vi "dll Main.vi"() -> ()   [LabVIEW 2018]
doc: "This template is for the Queued Message Handler design pattern.\n\nThe Event Handling Loop generates messages based on user interface actions.\n\nThe Message Handling Loop processes messages generated by the Event Handling Loop, or by other messages. The messages are string values, so new messages can be added easily to the Message Cases case structure in the Message Handling Loop. Each message cluster can also provide an optional value for Message Data, which is a variant that can be converted to whatever message-specific data is required."
uses:
  controls/dll UI Data.ctl
  support/Message Queue/dll Message Queue.lvlib
  <vilib>/Utility/error.llb/Error Cluster From Error Code.vi
  support/User Event - Stop/dll User Event - Stop.lvlib
  support/Message Queue/Enqueue Message (Single).vi
  <vilib>/ErrorRing/Error Ring.xnode
  C:/Users/booko/Desktop/ENABLE/UpDownCounter/bin/Debug/netstandard2.0/UpDownCounter.dll
  UpDownCounter/bin/Debug/netstandard2.0/UpDownCounter.dll
panel:
  out "Display <Replace Me>":string
  in  "Count Down":bool
  in  "Count Up":bool
  in  "Exit":bool
  # "These controls have associated \"Value Changed\" events configured in the Event Structure on the diagram.\n\nReplace them (and reconfigure the Event Structure) with the controls you need for your application."
  # "This template is for the Queued Message Handler design pattern.\n\nSee the block diagram for more information on how to use this template."
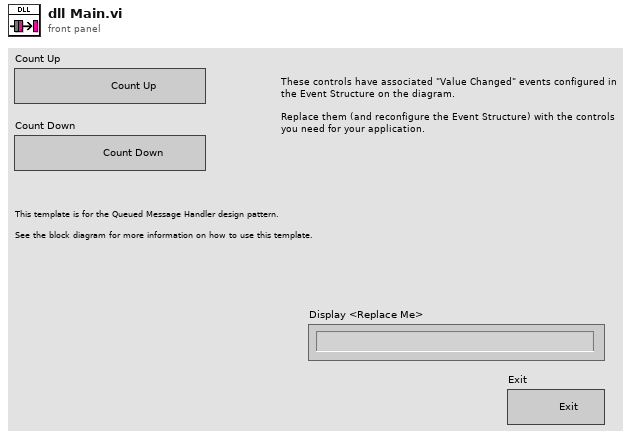
[diagram p1: front panel]
types:
  T1 = typedef "dll UI Data.ctl" = cluster{"Boolean <Replace Me>":bool, "String <Replace Me>":string, "Numeric <Replace Me>":dbl, "Do Something Ref":refnum<vi>, "Do Something Else Ref":refnum<vi>, "Data Display Ref":refnum<vi>, "Exit Button Ref":refnum<vi>, "UpDownCounterClass Reference":refnum<k24>}
  T2 = typedef "dll Message Queue.lvlib/All Message Queues.ctl" = cluster{"UI":refnum<queue>}
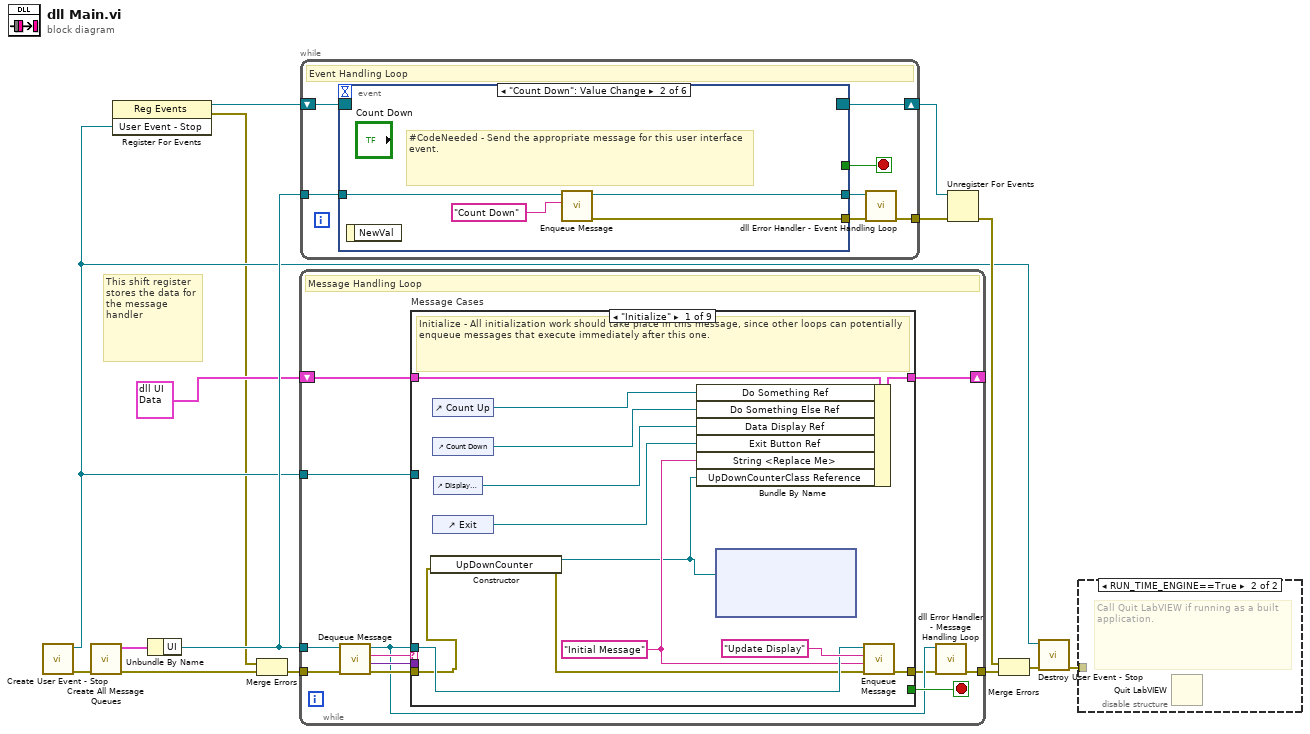
[diagram p0: block diagram]
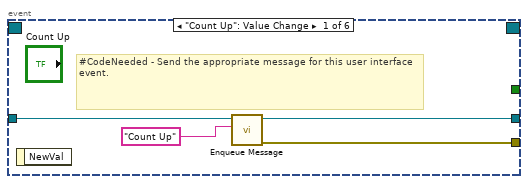
[diagram p3: hidden frame]
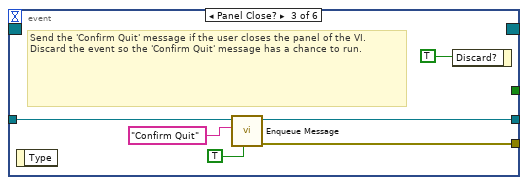
[diagram p4: hidden frame]
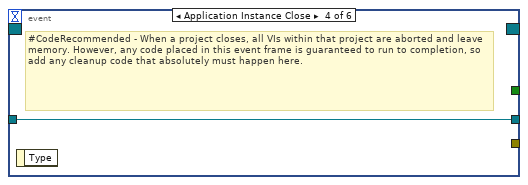
[diagram p5: hidden frame]
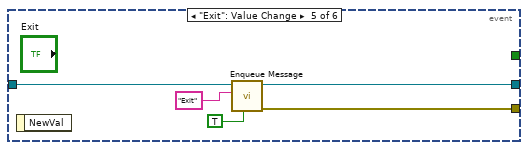
[diagram p6: hidden frame]
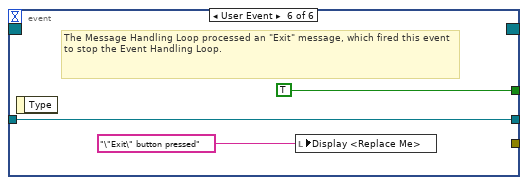
[diagram p7: hidden frame]
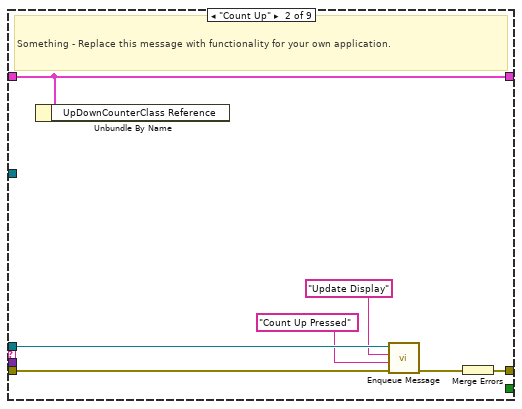
[diagram p8: hidden frame]
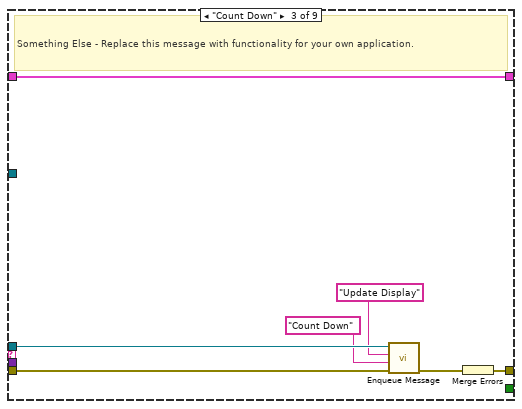
[diagram p9: hidden frame]
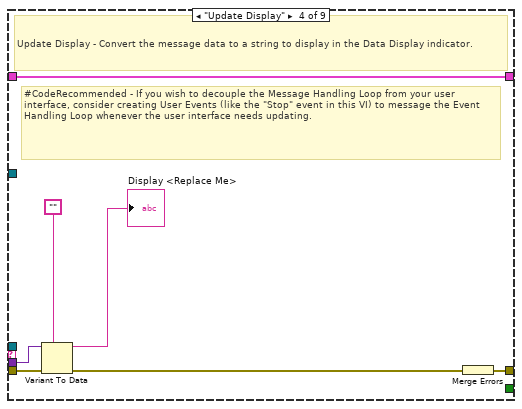
[diagram p10: hidden frame]
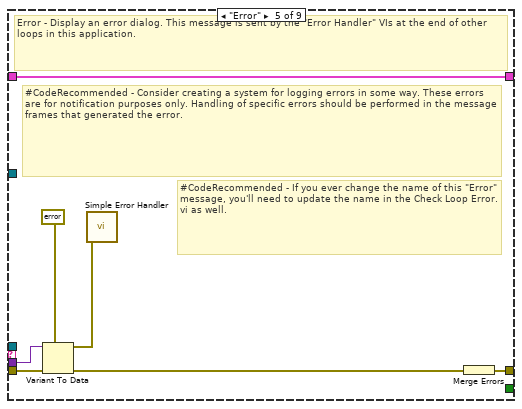
[diagram p11: hidden frame]
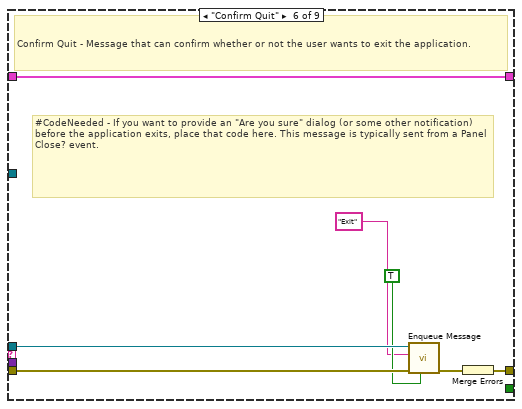
[diagram p12: hidden frame]
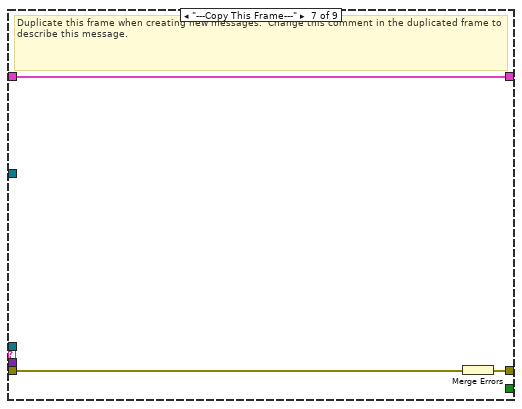
[diagram p13: hidden frame]
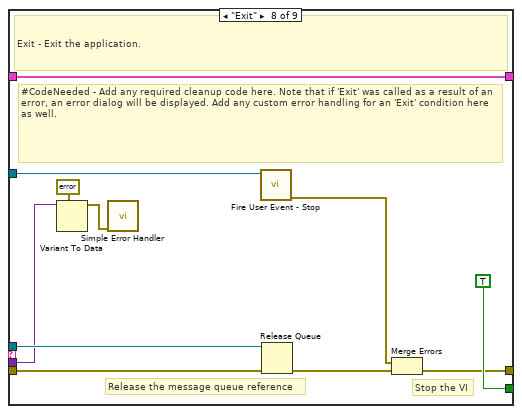
[diagram p14: hidden frame]
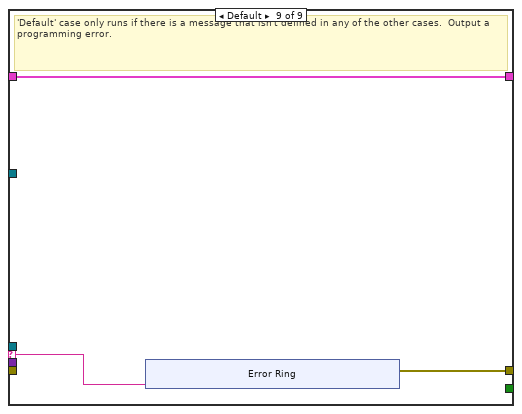
[diagram p15: hidden frame]
diagram:
  # "This shift register stores the data for the message handler"
  n1 = call "Create User Event - Stop.vi"() -> ("error out"=w11:errorcluster, "User Event - Stop"=w3:refnum<user-event>)  [unwired: 10 in]
  n2 = call "Create All Message Queues.vi"("error in (no error)"=w11) -> ("error out"=w15:errorcluster, "Message Queues out"=w14:T2)  [unwired: 9 in]
  n3 = register-events(w3) -> (reference out=w4:refnum<event-registration>, error out=w1:errorcluster)  [unwired: 2 in]
  n4 = Unbundle By Name(w14) -> ("UI"=w12:refnum<queue>)
  n5 = Merge Errors(w1, w15) -> (w2:errorcluster)
  n6 = while {
    tunnel: w12 -> [w19]
    shift-right: [w26] -> _
    shift-left: T1 {"Boolean <Replace Me>"=FALSE, "String <Replace Me>"="", "Numeric <Replace Me>"=0.0, "Do Something Ref"=refnum, "Do Something Else Ref"=refnum, "Data Display Ref"=refnum, "Exit Button Ref"=refnum, "UpDownCounterClass Reference"=refnum} ("Data Cluster") -> [w27]
    tunnel: w3 -> [w24]
    tunnel: w2 -> [w23]
    tunnel: [w17] -> w13
    stop <- w25 stop-if-true
    # "Message Handling Loop"
    n7 = call "Dequeue Message.vi"("error in (no error)"=w23, "Message Queue"=w19) -> ("error out"=w22:errorcluster, "Message Data"=w20:variant, "Message"=w21:string, "dup Message Queue"=w18:refnum<queue>)  [unwired: 6 in]
    n8 = case "Message Cases" shown="\"Initialize\"" w21 {
      selector: w21 -> [_ _ _ _ _ _ _ _ w90]
      tunnel: w18 -> [w32 w44 w50 _ _ w71 _ w89 _]
      tunnel: w22 -> [w30 w46 w52 w59 w68 w75 w78 w82 _]
      tunnel: [w40 w47 w53 w60 w62 w73 w76 w85 w91] -> w16
      tunnel: w27 -> [w39 w41 w54 w61 w67 w74 w77 w88 w92]
      tunnel: [w38 w41 w54 w61 w67 w74 w77 w88 w92] -> w26
      tunnel: [_ _ _ _ _ _ _ TRUE _] -> w25
      tunnel: w20 -> [_ _ _ w58 w66 _ _ w79 _]
      tunnel: w24 -> [_ _ _ _ _ _ _ w84 _]
      frame "Initialize" {
        w31 = "Initial Message" ("Initial Message")
        # "Initialize - All initialization work should take place in this message, since other loops can potentially enqueue messages that execute immediately after this one."
        n9 = constructor class="UpDownCounter"(error in=w30) -> (reference out=w28:refnum<k24>, error out=w29:errorcluster)  [unwired: 2 in, 1 out]
        n10 = control-ref of="Count Up"() -> (w37:refnum<vi>)
        n11 = control-ref of="Count Down"() -> (w36:refnum<vi>)
        n12 = control-ref of="Exit"() -> (w34:refnum<vi>)
        n13 = control-ref of="Display <Replace Me>"() -> (w35:refnum<vi>)
        n14 = Bundle By Name(cluster=w39, "Do Something Ref"=w37, "Do Something Else Ref"=w36, "Data Display Ref"=w35, "Exit Button Ref"=w34, "String <Replace Me>"=w31, "UpDownCounterClass Reference"=w28) -> (w38:T1)
        n15 = node(w28) -> ()  [unwired: 4 in, 2 out]
        n16 = call-poly "Enqueue Message.vi"("error in (no error)"=w29, "Message Data"=w31, "Message"="Update Display", "Message Queue"=w32) -> ("error out"=w40:errorcluster)  [unwired: 6 in, 1 out]
      }
      frame "Count Up" {
        # "Something - Replace this message with functionality for your own application."
        n17 = Unbundle By Name(w41) -> ()  [unwired: 1 out]
        n18 = call-poly "Enqueue Message.vi"("error in (no error)"=w46, "Message Data"="Count Up Pressed" ("\"Do Something\" button pressed"), "Message"="Update Display", "Message Queue"=w44) -> ("error out"=w45:errorcluster)  [unwired: 6 in, 1 out]
        n19 = Merge Errors(w45) -> (w47:errorcluster)
      }
      frame "Count Down" {
        # "Something Else - Replace this message with functionality for your own application."
        n20 = call-poly "Enqueue Message.vi"("error in (no error)"=w52, "Message Data"="Count Down" ("\"Do Something Else\" button pressed"), "Message"="Update Display", "Message Queue"=w50) -> ("error out"=w51:errorcluster)  [unwired: 6 in, 1 out]
        n21 = Merge Errors(w51) -> (w53:errorcluster)
      }
      frame "Update Display" {
        # "#CodeRecommended - If you wish to decouple the Message Handling Loop from your user interface, consider creating User Events (like the \"Stop\" event in this VI) to message the Event Handling Loop whenever the user interface needs updating."
        # "Update Display - Convert the message data to a string to display in the Data Display indicator."
        n22 = Variant To Data(error in=w59, type="", Variant=w58) -> (data=→"Display <Replace Me>":string, error out=w56:errorcluster)
        n23 = Merge Errors(w56) -> (w60:errorcluster)
      }
      frame "Error" {
        # "#CodeRecommended - If you ever change the name of this \"Error\" message, you'll need to update the name in the Check Loop Error.vi as well."
        # "#CodeRecommended - Consider creating a system for logging errors in some way. These errors are for notification purposes only. Handling of specific errors should be performed in the message frames that generated the error."
        # "Error - Display an error dialog. This message is sent by the \"Error Handler\" VIs at the end of other loops in this application."
        n24 = Variant To Data(error in=w68, type=errorcluster {"status"=FALSE, "code"=0, "source"=""} ("error constant"), Variant=w66) -> (data=w64:errorcluster, error out=w63:errorcluster)
        n25 = call <vilib>:"Simple Error Handler.vi"("error in (no error)"=w64) -> ()  [unwired: 4 in, 5 out]
        n26 = Merge Errors(w63) -> (w62:errorcluster)
      }
      frame "Confirm Quit" {
        # "#CodeNeeded - If you want to provide an \"Are you sure\" dialog (or some other notification) before the application exits, place that code here. This message is typically sent from a Panel Close? event."
        # "Confirm Quit - Message that can confirm whether or not the user wants to exit the application."
        n27 = call-poly "Enqueue Message.vi"("Priority Message? (F)"=TRUE, "error in (no error)"=w75, "Message"="Exit", "Message Queue"=w71) -> ("error out"=w72:errorcluster)  [unwired: 6 in, 1 out]
        n28 = Merge Errors(w72) -> (w73:errorcluster)
      }
      frame "---Copy This Frame---" {
        # "Duplicate this frame when creating new messages.  Change this comment in the duplicated frame to describe this message."
        n29 = Merge Errors(w78) -> (w76:errorcluster)
      }
      frame "Exit" {
        # "Stop the VI"
        # "Release the message queue reference"
        # "#CodeNeeded - Add any required cleanup code here. Note that if 'Exit' was called as a result of an error, an error dialog will be displayed. Add any custom error handling for an 'Exit' condition here as well."
        # "Exit - Exit the application."
        n30 = Variant To Data(type=errorcluster {"status"=FALSE, "code"=0, "source"=""} ("error constant"), Variant=w79) -> (data=w80:errorcluster)  [unwired: 1 in, 1 out]
        n31 = call <vilib>:"Simple Error Handler.vi"("error in (no error)"=w80) -> ()  [unwired: 4 in, 5 out]
        n32 = call "Fire User Event - Stop.vi"("User Event - Stop"=w84) -> ("error out"=w83:errorcluster)  [unwired: 10 in]
        n33 = Release Queue(queue=w89, error in (no error)=w82) -> (error out=w86:errorcluster)  [unwired: 1 in, 2 out]
        n34 = Merge Errors(w83, w86) -> (w85:errorcluster)
      }
      frame Default {
        # "'Default' case only runs if there is a message that isn't defined in any of the other cases.  Output a programming error."
        n35 = xnode "Error Ring"("parameter 0"=w90) -> ("error out"=w91:errorcluster)
      }
    }
    n36 = call "dll Error Handler - Message Handling Loop.vi"("error in (no error)"=w16, "Message Queue"=w18) -> ("dup error in"=w17:errorcluster)  [unwired: 8 in, 1 out]
  }
  n37 = while {
    tunnel: w12 -> [w106]
    shift-right: [w104] -> w8
    shift-left: w4 -> [w105]
    tunnel: [w100] -> w5
    stop <- w102 stop-if-true
    # "Event Handling Loop"
    n38 = event shown="[1] \"Count Down\": Value Change" {
      selector: w105 -> [_ _ _ _ _ _]
      dyn-events: [_ _ _ _ _ _] -> w104
      timeout: _ -> [_ _ _ _ _ _]
      tunnel: [_ _ _ _ _ TRUE ("Discard?")] -> w102
      tunnel: w106 -> [w110 w114 w119 w121 w126 w129]
      tunnel: [w107 w111 w118 _ w125 _] -> w103
      tunnel: [w109 w113 w117 w121 w124 w129] -> w101
      event "Count Up": Value Change {
        # "#CodeNeeded - Send the appropriate message for this user interface event."
        n39 = event-data() -> ()  [unwired: 1 in, 1 out]
        n40 = call-poly "Enqueue Message.vi"("Message"="Count Up", "Message Queue"=w110) -> ("error out"=w107:errorcluster, "dup Message Queue"=w109:refnum<queue>)  [unwired: 8 in]
      }
      event "Count Down": Value Change {
        # "#CodeNeeded - Send the appropriate message for this user interface event."
        n41 = event-data() -> ()  [unwired: 1 in, 1 out]
        n42 = call-poly "Enqueue Message.vi"("Message"="Count Down", "Message Queue"=w114) -> ("error out"=w111:errorcluster, "dup Message Queue"=w113:refnum<queue>)  [unwired: 8 in]
      }
      event Panel Close? {
        # "Send the 'Confirm Quit' message if the user closes the panel of the VI. Discard the event so the 'Confirm Quit' message has a chance to run."
        n43 = event-data() -> ()  [unwired: 1 in, 1 out]
        n44 = call-poly "Enqueue Message.vi"("Priority Message? (F)"=TRUE, "Message"="Confirm Quit", "Message Queue"=w119) -> ("error out"=w118:errorcluster, "dup Message Queue"=w117:refnum<queue>)  [unwired: 7 in]
        n45 = event-data("Discard?"=TRUE) -> ()  [unwired: 1 in, 1 out]
      }
      event Application Instance Close {
        # "#CodeRecommended - When a project closes, all VIs within that project are aborted and leave memory. However, any code placed in this event frame is guaranteed to run to completion, so add any cleanup code that absolutely must happen here."
        n46 = event-data() -> ()  [unwired: 1 in, 1 out]
      }
      event "Exit": Value Change {
        n47 = event-data() -> ()  [unwired: 1 in, 1 out]
        n48 = call-poly "Enqueue Message.vi"("Priority Message? (F)"=TRUE, "Message"="Exit", "Message Queue"=w126) -> ("error out"=w125:errorcluster, "dup Message Queue"=w124:refnum<queue>)  [unwired: 7 in]
      }
      event User Event {
        # "The Message Handling Loop processed an \"Exit\" message, which fired this event to stop the Event Handling Loop."
        n49 = event-data() -> ()  [unwired: 1 in, 1 out]
        n50 = local write "Display <Replace Me>"("\"Exit\" button pressed" ("VI Stopped")) -> ()
      }
    }
    n51 = call "dll Error Handler - Event Handling Loop.vi"("error in (no error)"=w103, "Message Queue"=w101) -> ("dup error in"=w100:errorcluster)  [unwired: 8 in, 1 out]
  }
  n52 = Unregister For Events(event registration refnum=w8, error in=w5) -> (error out=w9:errorcluster)
  n53 = Merge Errors(w9, w13) -> (w10:errorcluster)
  n54 = call "Destroy User Event - Stop.vi"("error in (no error)"=w10, "User Event - Stop"=w3) -> ("error out"=w6:errorcluster)  [unwired: 9 in]
  n55 = disable-structure shown="RUN_TIME_ENGINE==True" {
    disable-tunnel: w6 -> [_ _]
    frame condition #0 (active) {
    }
    frame condition #1 {
      # "Call Quit LabVIEW if running as a built application."
      n56 = Quit LabVIEW() -> ()  [unwired: 1 in]
    }
  }
